vi "Run.vi"(8 "error in (no error)":errorcluster, 10 "OTP Cluster Out":T1, 11 "Harmonics in":refnum<class "Harmonics.lvclass">) -> (0 "error out":errorcluster, 1 "Parameters":cluster{"Name":string, "Value":string}[](array[cluster]), 2 "Canceled":bool, 3 "Harmonics out":refnum<class "Harmonics.lvclass">)   [LabVIEW 2020, in "Harmonics.lvclass"]
doc: "This is the main test vi. It is here that the test is implemented."
uses:
  Harmonics.lvclass
  Controls/Run states.ctl
  Instruments/Spectrum Analyzer/Spectrum Analyzer.lvclass
  Measurement.lvclass
  Devices/Controls/Change setting mode enum.ctl
  Devices/PIC-device/PIC-Device.lvclass
  Controls/Loop order.ctl
  XML Handler/XML Handler.lvclass
  Support VI/Update parameters (single).vi
  Instruments/Power Supply/Power Supply.lvclass
  Support VI/Update parameters (array).vi
  Instruments/Digital Multimeter/Digital Multimeter.lvclass
  Devices/Device.lvclass
  Path Control/PathControl.lvclass
  Path Control/Paths.ctl
  Instruments/Power Meter/Power Meter.lvclass
  Instruments/Signal Generator/Signal Generator.lvclass
  C:/Sandbox/Git_Sandbox/WiSpry Test Framework source code (LV20)/WiSpry Test Framework/Measurements/Measurement.lvclass
  Controls/OTP_Cluster.ctl
panel:
  out "Power Meter reading (dBm)":dbl[](array[numeric])
  out "Parameters":string
  out "Current Power [dBm]":dbl
  out "Current Frequency [Hz]":dbl format="%#_6p"
  out "Progress":u8(slide) scale=0.0..100.0
  in  "Cancel Button":bool
  out "XY Graph":cluster{dbl[], dbl[]}[](graph)
  out "Estimated finish time":timestamp format="%<%X>T"
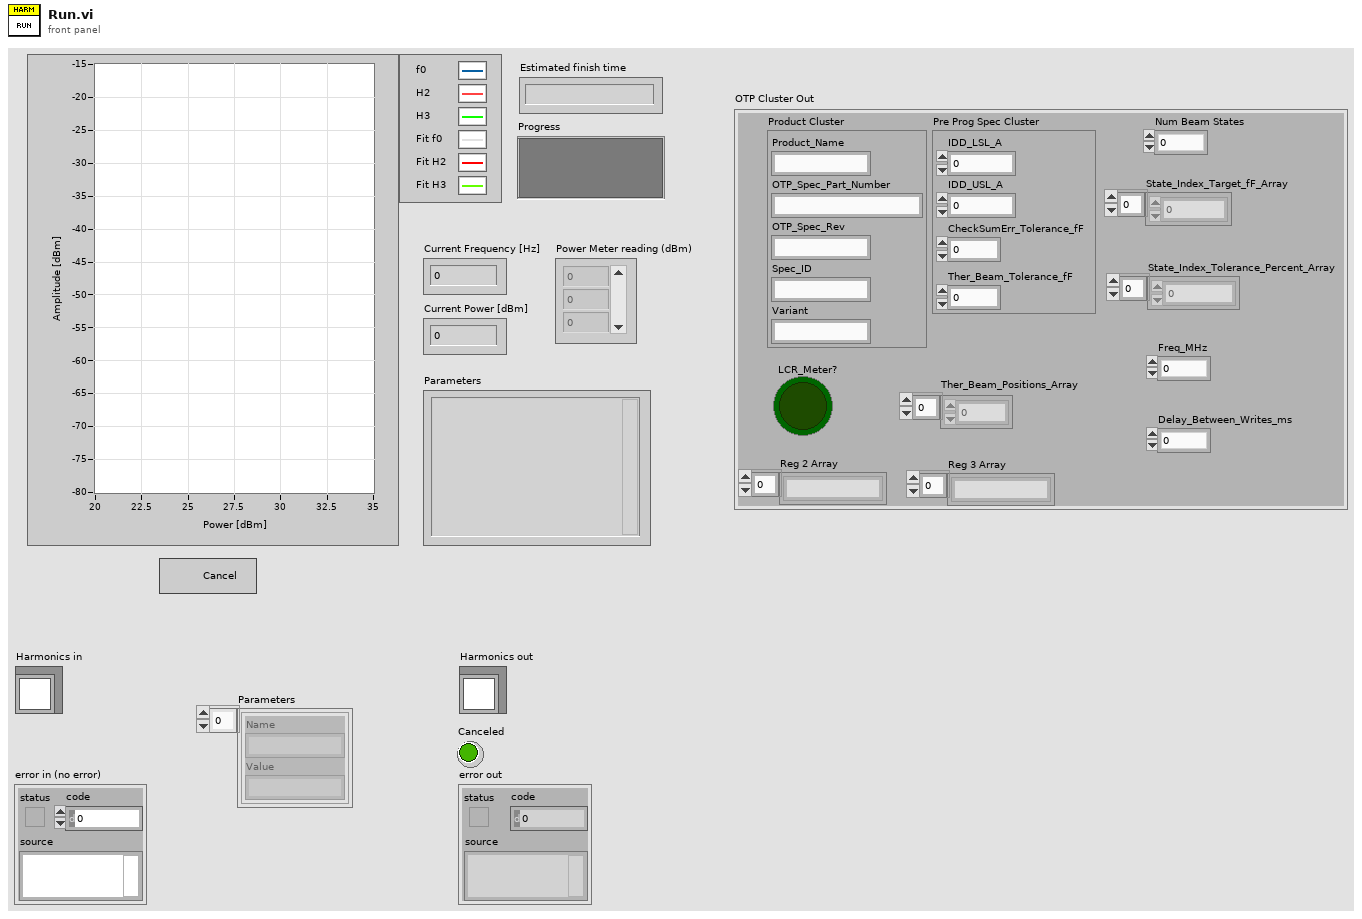
[diagram p1: front panel]
types:
  T1 = typedef "OTP_Cluster.ctl" = cluster{"Product Cluster":cluster{"Product_Name":string, "OTP_Spec_Part_Number":string, "OTP_Spec_Rev":string, "Spec_ID":string, "Variant":string}, "Pre Prog Spec Cluster":cluster{"IDD_LSL_A":dbl, "IDD_USL_A":dbl, "CheckSumErr_Tolerance_fF":dbl, "Ther_Beam_Tolerance_fF":dbl}, "LCR_Meter?":bool, "Reg 2 Array":string[], "Reg 3 Array":string[], "Num Beam States":i32, "State_Index_Target_fF_Array":dbl[], "State_Index_Tolerance_Percent_Array":dbl[], "Freq_MHz":dbl, "Delay_Between_Writes_ms":i32, "Ther_Beam_Positions_Array":i8[]}
  T2 = typedef "Harmonics.lvclass/Loop order.ctl" = enum16{"Device -> Power -> Frequency", "Device -> Frequency -> Power"}
  T3 = typedef "Harmonics.lvclass/Run states.ctl" = enum16{"Init", "Set Device", "Set Power", "Set Frequency", "Read Environment", "Measure", "Done"}
  T4 = typedef "PIC-Device.lvclass/Change setting mode enum.ctl" = enum16{"Init", "Next", "Reset"}
  T5 = typedef "PathControl.lvclass/Paths.ctl" = enum16{"SigGen 1 -> DUT", "SigGen 2 -> DUT", "SigGen 1 -> PM 1", "SigGen 1 -> PM 2", "DUT -> SA", "DUT -> PM 2", "VSG -> DUT", "SigGen 2 -> PM 1", "SigGen 2 -> PM 2"}
  T6 = typedef "Harmonics.lvclass/Config info.ctl" = cluster{"RBW":dbl, "VBW ":dbl, "Number of Averages":i32, "Average On":bool, "Symbols":i32[], "All Harm":bool, "Loop order":T2, "Power Window":dbl, "Frequency (MHz)":string, "Power (dBm)":string, "PM for power leveling":u8, "Zero span":bool, "Stop level":dbl}
  T7 = typedef "XML Handler.lvclass/Result Cluster.ctl" = cluster{"Name":string, "Value":string}
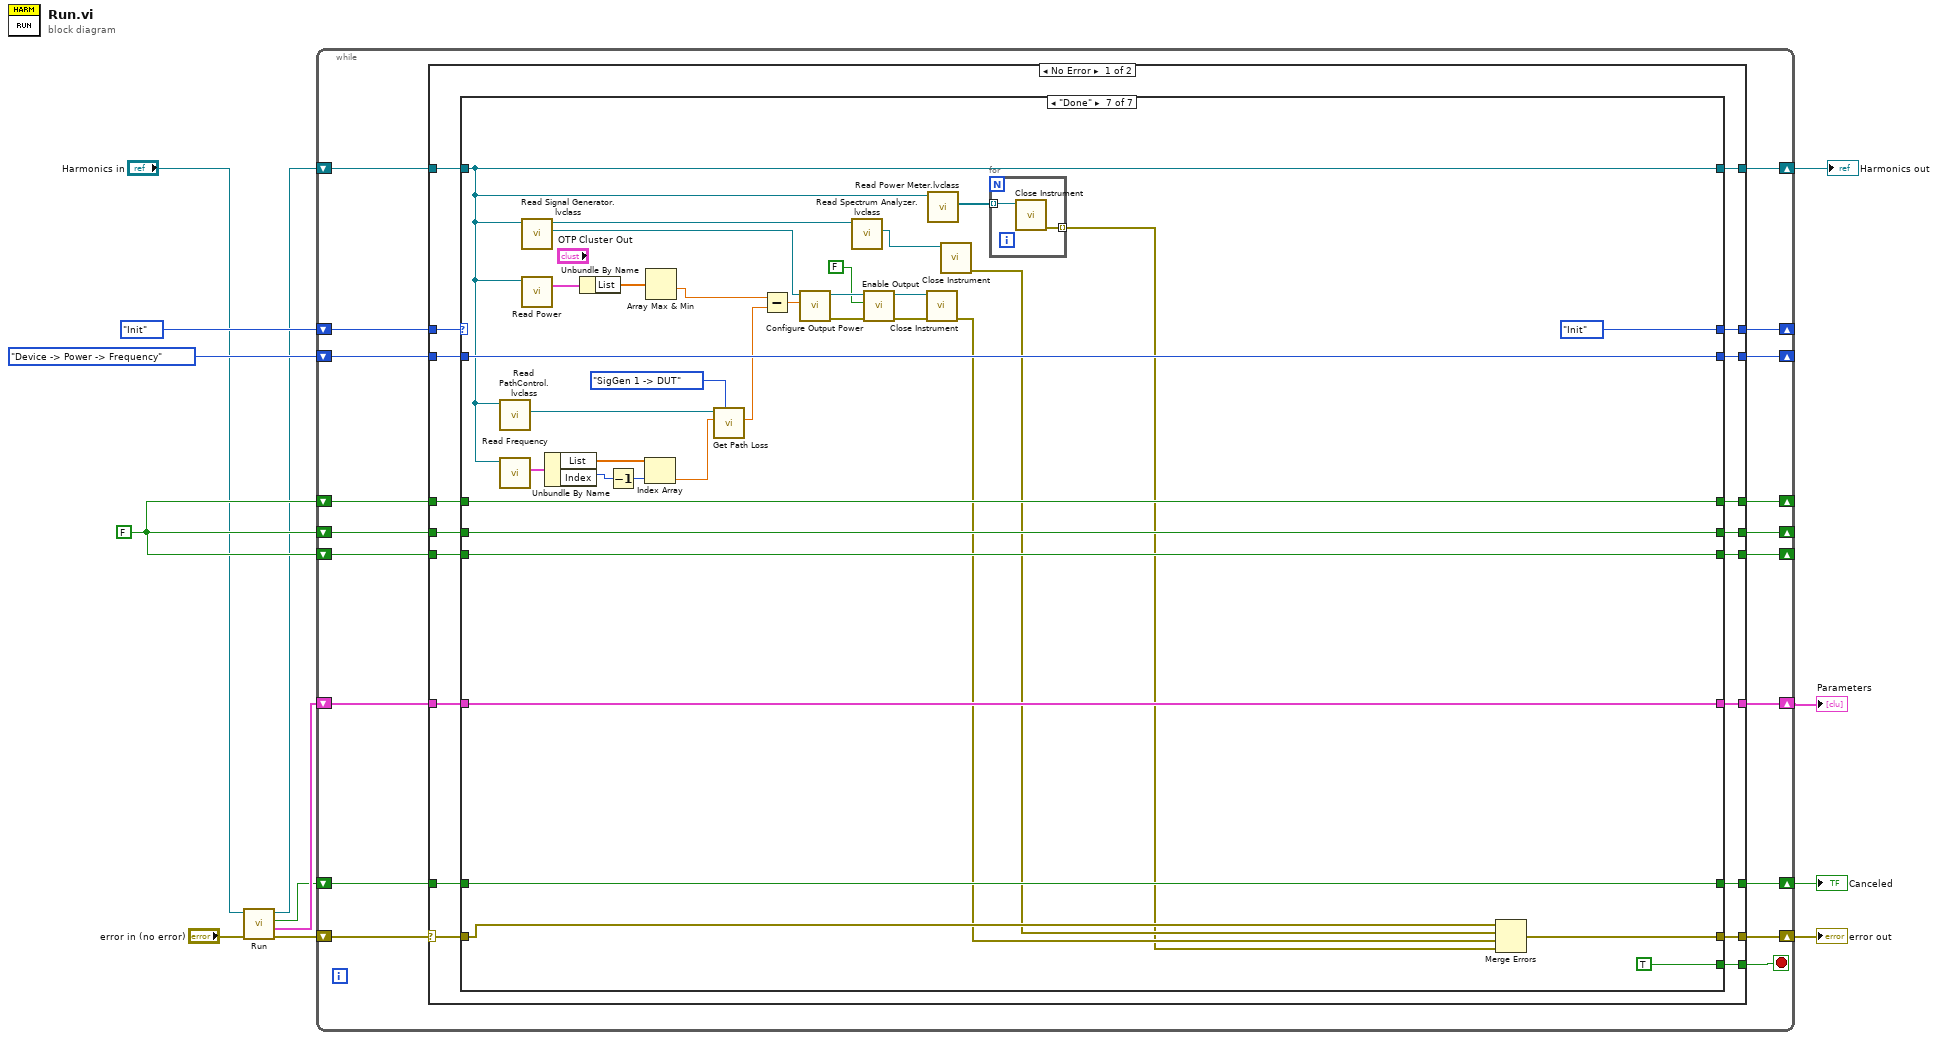
[diagram p0: block diagram]
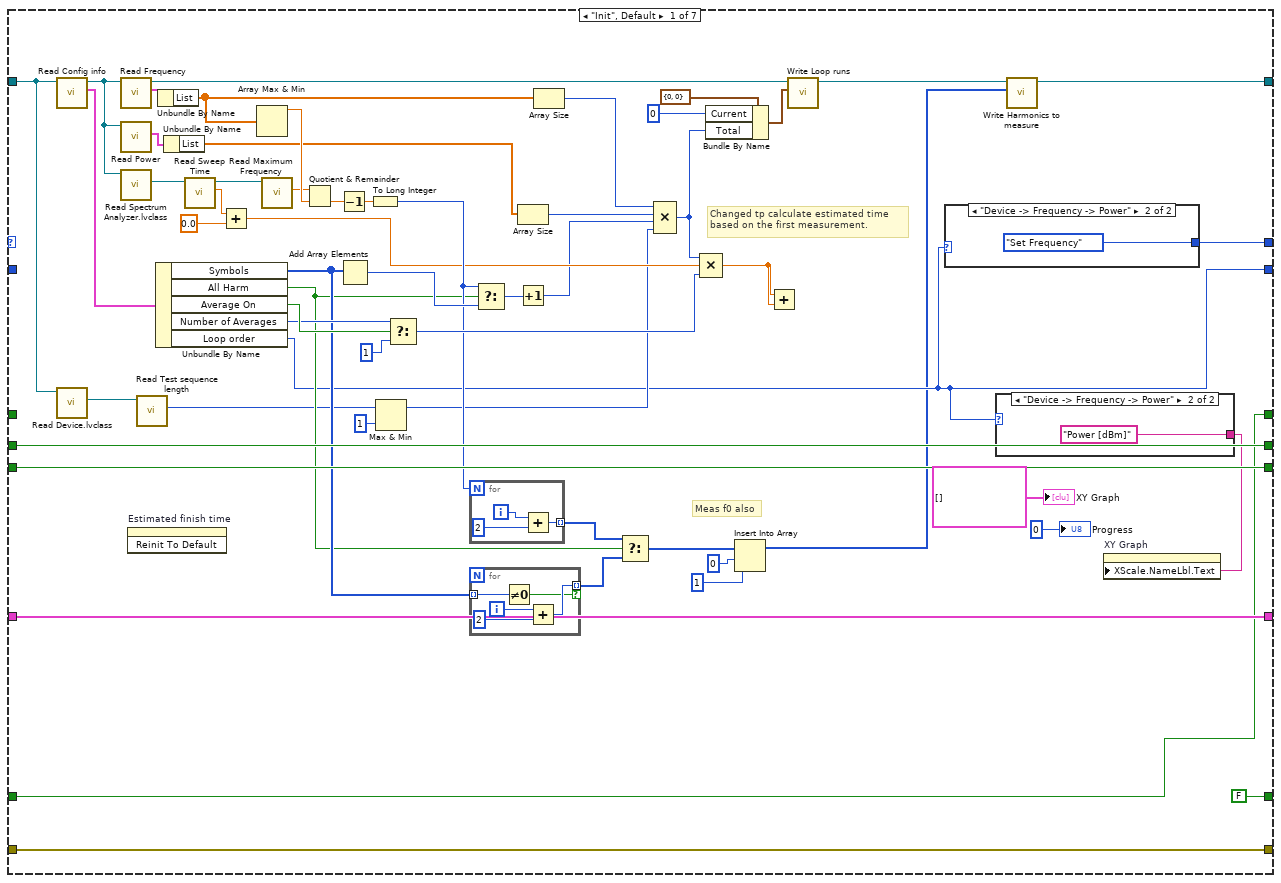
[diagram p2: hidden frame]
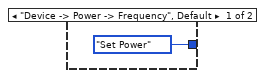
[diagram p3: hidden frame]
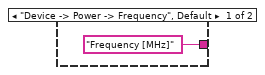
[diagram p4: hidden frame]
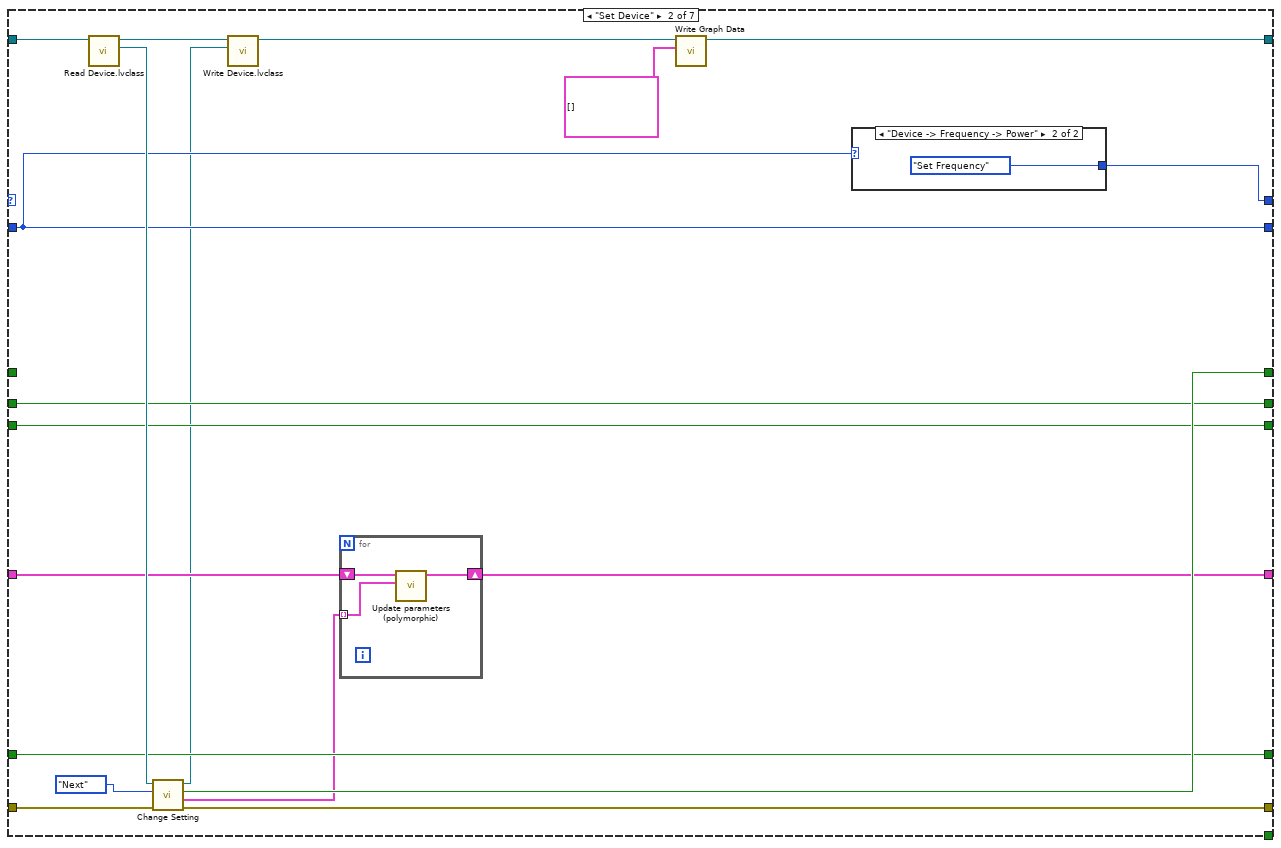
[diagram p5: hidden frame]
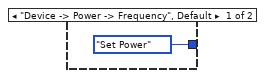
[diagram p6: hidden frame]
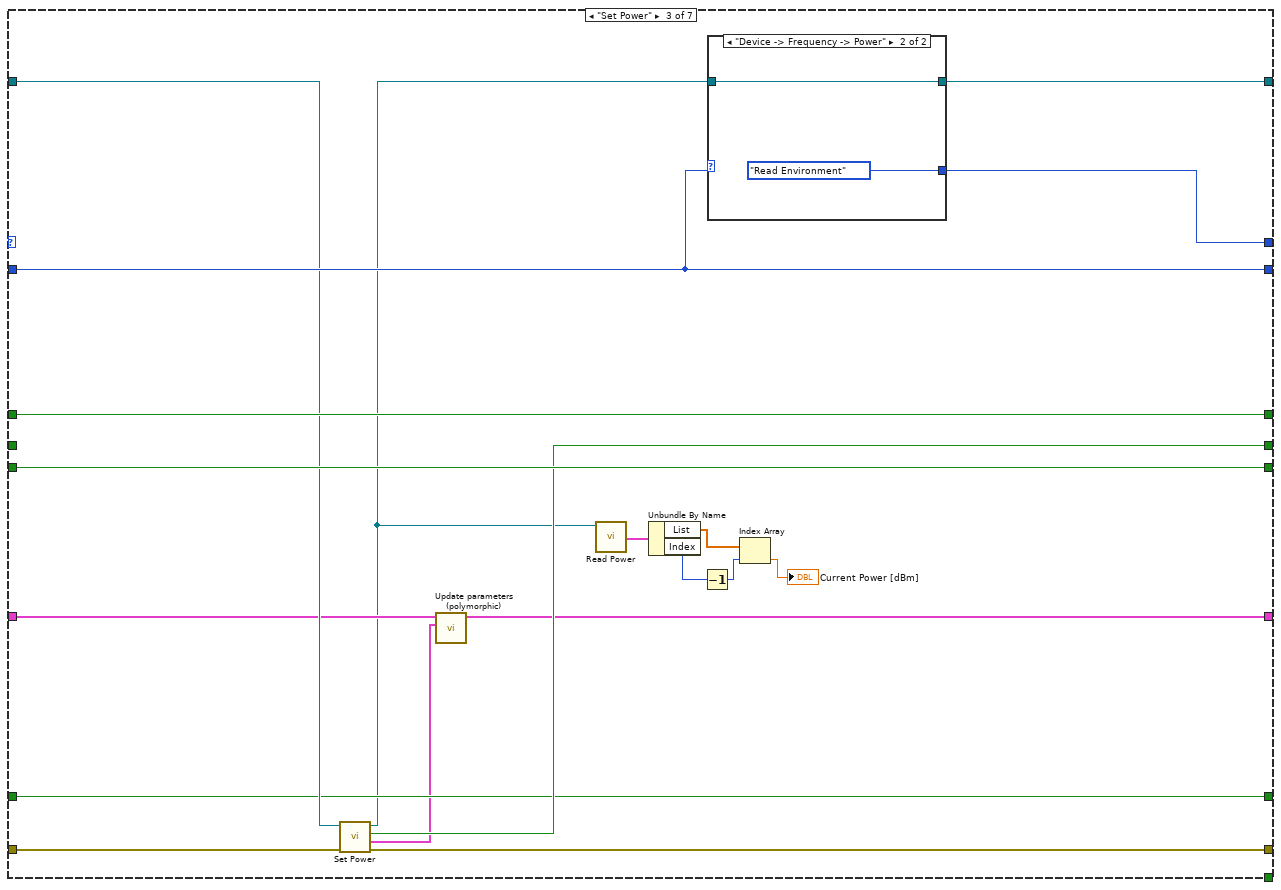
[diagram p7: hidden frame]
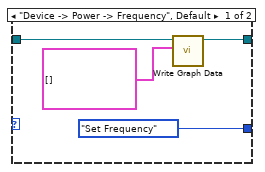
[diagram p8: hidden frame]
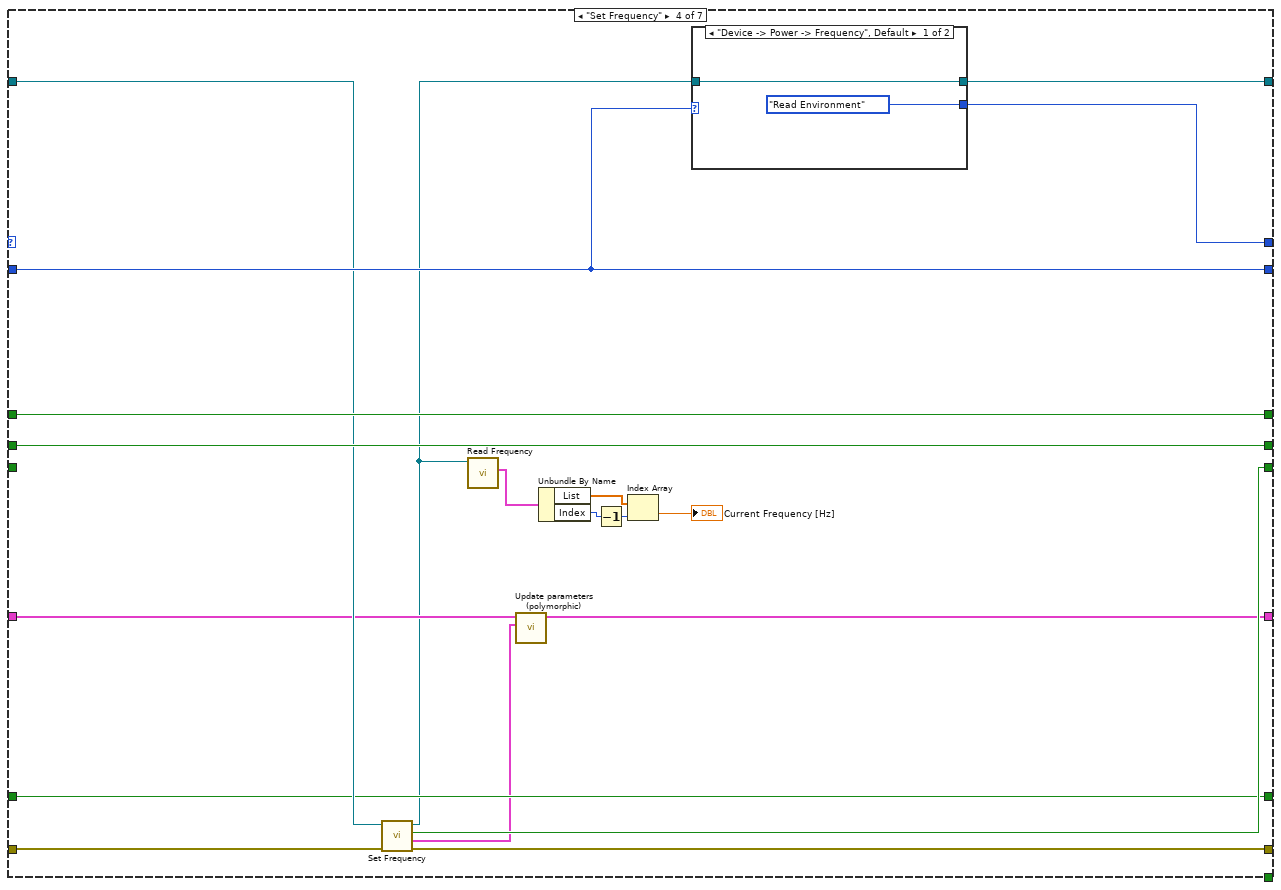
[diagram p9: hidden frame]
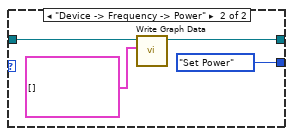
[diagram p10: hidden frame]
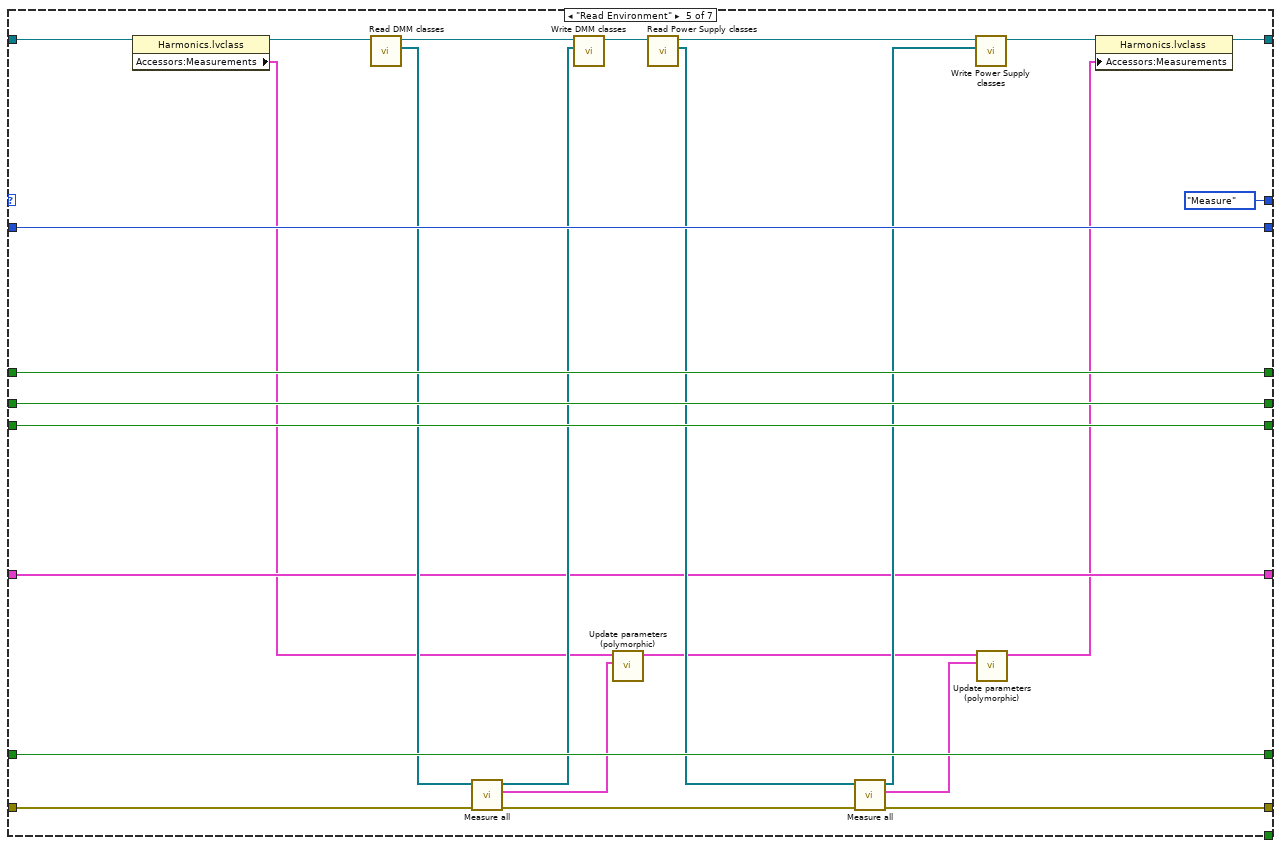
[diagram p11: hidden frame]
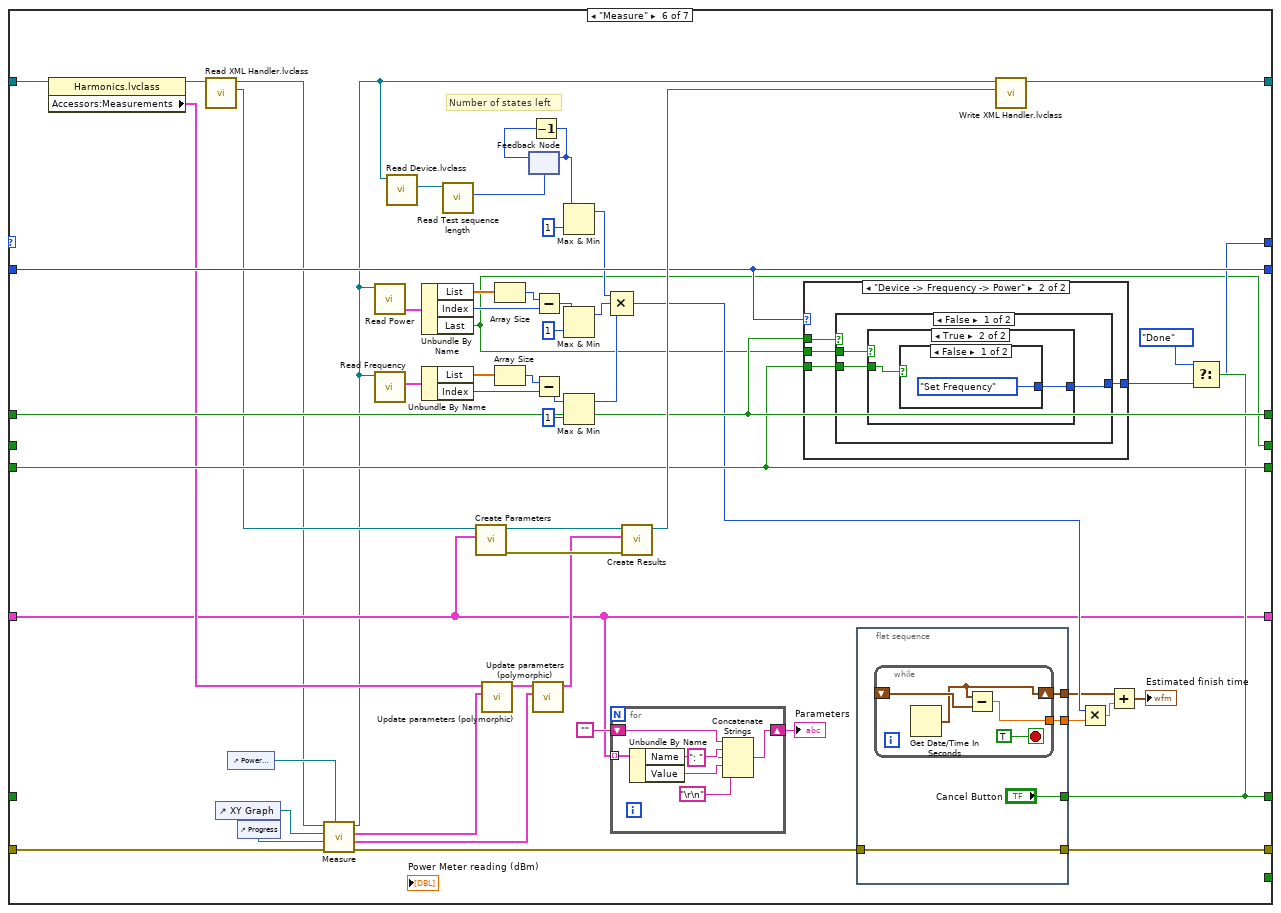
[diagram p12: hidden frame]
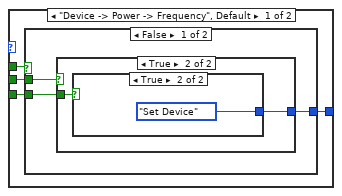
[diagram p13: hidden frame]
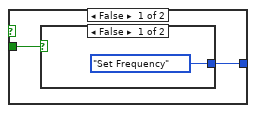
[diagram p14: hidden frame]
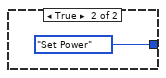
[diagram p15: hidden frame]
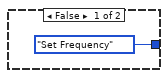
[diagram p16: hidden frame]
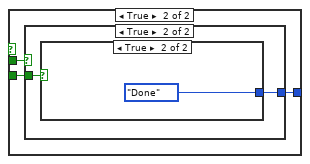
[diagram p17: hidden frame]
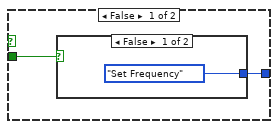
[diagram p18: hidden frame]
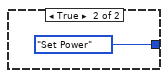
[diagram p19: hidden frame]
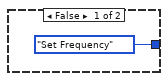
[diagram p20: hidden frame]
diagram:
  w10 = FALSE
  n1 = call-parent "Run.vi"("error in (no error)"="error in (no error)", "Measurements in"="Harmonics in") -> ("error out"=w5:errorcluster, "Parameters"=w3:cluster{"Name":string, "Value":string}[], "Canceled"=w2:bool, "Measurements out"=w1:refnum<class "Harmonics.lvclass">)  [unwired: 5 in, 1 out]
  n2 = while {
    shift-right: [w29] -> w12
    shift-left: w5 -> [w15]
    shift-right: [w31] -> w13
    shift-left: w1 -> [w14]
    shift-right: [w26] -> _
    shift-left: Run_states."Init" ("Run states") -> [w32]
    shift-right: [w28] -> _
    shift-left: w10 -> [w27]
    shift-right: [w25] -> _
    shift-left: Loop_order."Device -> Power -> Frequency" ("Loop order") -> [w24]
    shift-right: [w21] -> _
    shift-left: w10 -> [w23]
    shift-right: [w20] -> _
    shift-left: w10 -> [w22]
    shift-right: [w19] -> w8
    shift-left: w2 -> [w18]
    shift-right: [w16] -> w7
    shift-left: w3 -> [w17]
    stop <- w30 stop-if-true
    n3 = case shown="No Error" w15 {
      selector: w15 -> [w48 w376]
      tunnel: w14 -> [w51 w377]
      tunnel: w32 -> [w50 _]
      tunnel: [w49 w377] -> w31
      tunnel: [w47 TRUE] -> w30
      tunnel: [w46 w376] -> w29
      tunnel: [w45 _] -> w28
      tunnel: w27 -> [w44 _]
      tunnel: [w43 _] -> w26
      tunnel: [w42 _] -> w25
      tunnel: w24 -> [w41 _]
      tunnel: w23 -> [w40 _]
      tunnel: w22 -> [w39 _]
      tunnel: [w38 _] -> w21
      tunnel: [w37 _] -> w20
      tunnel: [w36 _] -> w19
      tunnel: w18 -> [w35 _]
      tunnel: w17 -> [w34 w375]
      tunnel: [w33 w375] -> w16
      frame No Error {
        n4 = case shown="\"Done\"" w50 {
          tunnel: w51 -> [w94 w139 w158 w183 w199 w223 w342]
          tunnel: [w83 w128 w155 w180 w200 w274 w342] -> w49
          tunnel: w48 -> [w69 w136 w159 w184 w205 w238 w360]
          tunnel: [_ _ _ _ _ _ TRUE] -> w47
          tunnel: [w69 w125 w154 w179 w204 w272 w357] -> w46
          tunnel: [w60 w135 w163 w188 w220 w270 w371] -> w45
          tunnel: w44 -> [_ _ w163 w188 w220 w270 w371]
          tunnel: [w62 w131 w161 w186 Run_states."Measure" ("Run states") w265 Run_states."Init" ("Run states")] -> w43
          tunnel: [w61 w132 w162 w187 w219 w271 w372] -> w42
          tunnel: w41 -> [_ w132 w162 w187 w219 w271 w372]
          tunnel: w40 -> [w90 w134 _ w185 w218 _ w370]
          tunnel: w39 -> [w89 w133 w160 _ w217 w269 w369]
          tunnel: [w90 w134 w157 w185 w218 w221 w370] -> w38
          tunnel: [w89 w133 w160 w182 w217 w269 w369] -> w37
          tunnel: [FALSE ("Last setting") w130 w156 w181 w216 w268 w366] -> w36
          tunnel: w35 -> [w60 w130 w156 w181 w216 _ w366]
          tunnel: w34 -> [w73 w124 w153 w178 w197 w225 w365]
          tunnel: [w73 w122 w152 w177 w197 w225 w365] -> w33
          frame "Init", Default {
            # "Changed tp calculate estimated time \nbased on the first measurement."
            # "Meas f0 also"
            n5 = call "Read Config info.vi"("Harmonics in"=w94) -> ("Config info"=w107:T6, "Harmonics out"=w108:refnum<class "Harmonics.lvclass">)  [unwired: 9 in]
            n6 = call "Read Device.lvclass.vi"("Measurements in"=w94) -> ("Device.lvclass"=w91:refnum<class "Device.lvclass">)  [unwired: 9 in, 1 out]
            n7 = call "Read Frequency.vi"("Harmonics in"=w108) -> ("Frequency"=w82:cluster{"List":dbl[], "Index":i32, "Last":bool}, "Harmonics out"=w78:refnum<class "Harmonics.lvclass">)  [unwired: 9 in]
            n8 = call "Read Power.vi"("Harmonics in"=w108) -> ("Power"=w80:cluster{"List":dbl[], "Index":i32, "Last":bool})  [unwired: 9 in, 1 out]
            n9 = call "Read Spectrum Analyzer.lvclass.vi"("Harmonics in"=w108) -> ("Spectrum Analyzer.lvclass"=w105:refnum<class "Spectrum Analyzer.lvclass">)  [unwired: 9 in, 1 out]
            n10 = invoke on="Estimated finish time" class="AbsTime (strict)" method="Reinit To Default"() -> ()  [unwired: 3 in, 3 out]
            n11 = call-dynamic "Read Test sequence length.vi"("Device in"=w91) -> ("Test sequence length"=w65:i32)  [unwired: 8 in, 2 out]
            n12 = Unbundle By Name(w107) -> ("Symbols"=w87:i32[], "All Harm"=w84:bool, "Average On"=w99:bool, "Number of Averages"=w98:i32, "Loop order"=w61:T2)
            n13 = Unbundle By Name(w82) -> ("List"=w81:dbl[])
            n14 = Unbundle By Name(w80) -> ("List"=w79:dbl[])
            n15 = call "Read Sweep Time.vi"("Spectrum Analyzer in"=w105) -> ("Sweep Time"=w100:dbl, "Spectrum Analyzer out"=w104:refnum<class "Spectrum Analyzer.lvclass">)  [unwired: 9 in]
            n16 = Add(x=w100, y=0.0) -> (x+y=w67:dbl)
            n17 = Array Max & Min(array=w81) -> (max value=w103:dbl)  [unwired: 3 out]
            n18 = call "Read Maximum Frequency.vi"("Spectrum Analyzer in"=w104) -> ("Maximum Frequency"=w102:dbl)  [unwired: 9 in, 1 out]
            n19 = Quotient & Remainder(x=w102, y=w103) -> (floor(x/y)=w101:dbl)  [unwired: 1 out]
            n20 = Decrement(x=w101) -> (x-1=w95:dbl)
            n21 = Add Array Elements(numeric array=w87) -> (sum=w106:i32)
            n22 = To Long Integer(number=w95) -> (32bit integer=w88:i32)
            n23 = Max & Min(x=w65, y=1) -> (max(x,y)=w64:i32)  [unwired: 1 out]
            n24 = Select(t=w98, s=w99, f=1) -> (s? t:f=w96:i32)
            n25 = for {
              N: w88 -> [_]
              tunnel: [w118] -> w86 mode=indexing
              i -> [w120]
              n26 = Add(x=w120, y=2) -> (x+y=w118:i32)
            }
            n27 = for {
              tunnel: w87 -> [w114] mode=indexing
              tunnel: [w115] -> w85 mode=indexing if=w113
              i -> [w117]
              n28 = Not Equal To 0?(x=w114) -> (x != 0?=w113:bool)
              n29 = Add(x=w117, y=2) -> (x+y=w115:i32)
            }
            n30 = Select(t=w88, s=w84, f=w106) -> (s? t:f=w54:i32)
            n31 = Array Size(array=w79) -> (size(s)=w92:i32)
            n32 = Increment(x=w54) -> (x+1=w53:i32)
            n33 = Array Size(array=w81) -> (size(s)=w93:i32)
            n34 = Select(t=w86, s=w84, f=w85) -> (s? t:f=w58:i32[])
            n35 = Compound Arithmetic op=MULTIPLY(w93, w92, w53, w64) -> (w74:i32)
            n36 = Compound Arithmetic op=MULTIPLY(w74, w67, w96) -> (w52:dbl)
            n37 = Bundle By Name(cluster=cluster{"Current":u32, "Total":u32} {"Current"=0, "Total"=0} ("Loop runs"), "Current"=u32 0, "Total"=w74) -> (w75:cluster{"Current":u32, "Total":u32})
            n38 = Insert Into Array(array=w58, index=0, new element=1 ("new element/subarray")) -> (w57:i32[])
            n39 = Add(x=w52, y=w52) -> ()  [unwired: 1 out]
            n40 = call "Write Loop runs.vi"("Loop runs"=w75, "Measurements in"=w78) -> ("Measurements out"=w68:refnum<class "Harmonics.lvclass">)  [unwired: 9 in]
            n41 = case shown="\"Device -> Frequency -> Power\"" w61 {
              tunnel: [Run_states."Set Power" ("Run states") Run_states."Set Frequency" ("Run states")] -> w62
              frame "Device -> Power -> Frequency", Default {
              }
              frame "Device -> Frequency -> Power" {
              }
            }
            n42 = case shown="\"Device -> Frequency -> Power\"" w61 {
              tunnel: ["Frequency [MHz]" "Power [dBm]"] -> w70
              frame "Device -> Power -> Frequency", Default {
              }
              frame "Device -> Frequency -> Power" {
              }
            }
            n43 = call "Write Harmonics to measure.vi"("Harmonics to measure"=w57, "Harmonics in"=w68) -> ("Harmonics out"=w83:refnum<class "Harmonics.lvclass">)  [unwired: 9 in]
            n44 = property on="XY Graph" class="XYGraph (strict)"("XScale.NameLbl.Text"=w70) -> ()  [unwired: 2 in, 2 out]
            "XY Graph" <- cluster{dbl[], dbl[]}[] [] ("XY Graph")
            "Progress" <- u8 0 ("Progress")
          }
          frame "Set Device" {
            n45 = call "Read Device.lvclass.vi"("Measurements in"=w139) -> ("Device.lvclass"=w138:refnum<class "Device.lvclass">, "Measurements out"=w129:refnum<class "Harmonics.lvclass">)  [unwired: 9 in]
            n46 = call-dynamic "Change Setting.vi"("error in (no error)"=w136, "Change setting mode"=Change_setting_mode_enum."Next", "Device in"=w138) -> ("error out"=w125:errorcluster, "Changes"=w123:cluster{"Name":string, "Value":string}[], "Last setting"=w135:bool, "Device out"=w121:refnum<class "Device.lvclass">)  [unwired: 5 in]
            n47 = call "Write Device.lvclass.vi"("Device.lvclass"=w121, "Measurements in"=w129) -> ("Measurements out"=w126:refnum<class "Harmonics.lvclass">)  [unwired: 9 in]
            n48 = for {
              shift-right: [w141] -> w122
              shift-left: w124 -> [w142]
              tunnel: w123 -> [w140] mode=indexing
              n49 = call-poly "Update parameters (polymorphic).vi"("New Parameter"=w140, "Parameters"=w142) -> ("Parameters Out"=w141:cluster{"Name":string, "Value":string}[])  [unwired: 9 in]
            }
            n50 = call "Write Graph Data.vi"("Graph Data"=cluster{"Array":dbl[], "Array":dbl[]}[] [], "Harmonics in"=w126) -> ("Harmonics out"=w128:refnum<class "Harmonics.lvclass">)  [unwired: 9 in]
            n51 = case shown="\"Device -> Frequency -> Power\"" w132 {
              tunnel: [Run_states."Set Power" ("Run states") Run_states."Set Frequency" ("Run states")] -> w131
              frame "Device -> Power -> Frequency", Default {
              }
              frame "Device -> Frequency -> Power" {
              }
            }
          }
          frame "Set Power" {
            n52 = call "Set Power.vi"("error in (no error)"=w159, "Harmonics in"=w158) -> ("error out"=w154:errorcluster, "Parameter"=w151:cluster{"Name":string, "Value":string}, "Last Power?"=w157:bool, "Harmonics out"=w150:refnum<class "Harmonics.lvclass">)  [unwired: 6 in]
            n53 = call-poly "Update parameters (polymorphic).vi"("New Parameter"=w151, "Parameters"=w153) -> ("Parameters Out"=w152:cluster{"Name":string, "Value":string}[])  [unwired: 9 in]
            n54 = call "Read Power.vi"("Harmonics in"=w150) -> ("Power"=w149:cluster{"List":dbl[], "Index":i32, "Last":bool})  [unwired: 9 in, 1 out]
            n55 = Unbundle By Name(w149) -> ("List"=w147:dbl[], "Index"=w145:i32)
            n56 = Decrement(x=w145) -> (x-1=w146:i32)
            n57 = case shown="\"Device -> Frequency -> Power\"" w162 {
              tunnel: [Run_states."Set Frequency" ("Run states") Run_states."Read Environment" ("Run states")] -> w161
              tunnel: w150 -> [w166 w168]
              tunnel: [w165 w168] -> w155
              frame "Device -> Power -> Frequency", Default {
                n58 = call "Write Graph Data.vi"("Graph Data"=cluster{"Array":dbl[], "Array":dbl[]}[] [], "Harmonics in"=w166) -> ("Harmonics out"=w165:refnum<class "Harmonics.lvclass">)  [unwired: 9 in]
              }
              frame "Device -> Frequency -> Power" {
              }
            }
            n59 = Index Array(array=w147, index=w146) -> (element=→"Current Power [dBm]":dbl)
          }
          frame "Set Frequency" {
            n60 = call "Set Frequency.vi"("error in (no error)"=w184, "Harmonics in"=w183) -> ("error out"=w179:errorcluster, "Parameter"=w176:cluster{"Name":string, "Value":string}, "Last Frequency?"=w182:bool, "Harmonics out"=w175:refnum<class "Harmonics.lvclass">)  [unwired: 6 in]
            n61 = call "Read Frequency.vi"("Harmonics in"=w175) -> ("Frequency"=w174:cluster{"List":dbl[], "Index":i32, "Last":bool})  [unwired: 9 in, 1 out]
            n62 = call-poly "Update parameters (polymorphic).vi"("New Parameter"=w176, "Parameters"=w178) -> ("Parameters Out"=w177:cluster{"Name":string, "Value":string}[])  [unwired: 9 in]
            n63 = Unbundle By Name(w174) -> ("List"=w173:dbl[], "Index"=w172:i32)
            n64 = Decrement(x=w172) -> (x-1=w171:i32)
            n65 = Index Array(array=w173, index=w171) -> (element=→"Current Frequency [Hz]":dbl)
            n66 = case shown="\"Device -> Power -> Frequency\", Default" w187 {
              tunnel: [Run_states."Read Environment" ("Run states") Run_states."Set Power" ("Run states")] -> w186
              tunnel: [w189 w192] -> w180
              tunnel: w175 -> [w189 w193]
              frame "Device -> Power -> Frequency", Default {
              }
              frame "Device -> Frequency -> Power" {
                n67 = call "Write Graph Data.vi"("Graph Data"=cluster{"Array":dbl[], "Array":dbl[]}[] [], "Harmonics in"=w193) -> ("Harmonics out"=w192:refnum<class "Harmonics.lvclass">)  [unwired: 9 in]
              }
            }
          }
          frame "Read Environment" {
            n68 = property class="Harmonics.lvclass"(reference=w199) -> (reference out=w198:refnum<class "Harmonics.lvclass">, "Accessors:Measurements"=w196:cluster{"Name":string, "Value":string}[])  [unwired: 1 in, 1 out]
            n69 = call-dynamic "Read DMM classes.vi"("Measurements in"=w198) -> ("DMM classes"=w210:refnum<class "Digital Multimeter.lvclass">[], "Measurements out"=w215:refnum<class "Harmonics.lvclass">)  [unwired: 9 in]
            n70 = call "Measure all.vi"("error in (no error)"=w205, "Digital Multimeters in"=w210) -> ("error out"=w208:errorcluster, "Measurements"=w207:T7[], "Digital Multimeters out"=w209:refnum<class "Digital Multimeter.lvclass">[])  [unwired: 5 in, 2 out]
            n71 = call-dynamic "Write DMM classes.vi"("DMM classes"=w209, "Measurements in"=w215) -> ("Measurements out"=w212:refnum<class "Harmonics.lvclass">)  [unwired: 9 in]
            n72 = call-poly "Update parameters (polymorphic).vi"("New Parameters"=w207, "Parameters"=w196) -> ("Parameters Out"=w206:cluster{"Name":string, "Value":string}[])  [unwired: 9 in]
            n73 = call-dynamic "Read Power Supply classes.vi"("Measurements in"=w212) -> ("Power Supply classes"=w214:refnum<class "Power Supply.lvclass">[], "Measurements out"=w202:refnum<class "Harmonics.lvclass">)  [unwired: 9 in]
            n74 = call "Measure all.vi"("error in (no error)"=w208, "Power Supplies in"=w214) -> ("error out"=w204:errorcluster, "Measurements"=w211:T7[], "Power Supplies out"=w213:refnum<class "Power Supply.lvclass">[])  [unwired: 5 in, 2 out]
            n75 = call-dynamic "Write Power Supply classes.vi"("Power Supply classes"=w213, "Measurements in"=w202) -> ("Measurements out"=w201:refnum<class "Harmonics.lvclass">)  [unwired: 9 in]
            n76 = call-poly "Update parameters (polymorphic).vi"("New Parameters"=w211, "Parameters"=w206) -> ("Parameters Out"=w195:cluster{"Name":string, "Value":string}[])  [unwired: 9 in]
            n77 = property class="Harmonics.lvclass"(reference=w201, "Accessors:Measurements"=w195) -> (reference out=w200:refnum<class "Harmonics.lvclass">)  [unwired: 1 in, 1 out]
          }
          frame "Measure" {
            # "Number of states left"
            n78 = property class="Harmonics.lvclass"(reference=w223) -> (reference out=w260:refnum<class "Harmonics.lvclass">, "Accessors:Measurements"=w259:cluster{"Name":string, "Value":string}[])  [unwired: 1 in, 1 out]
            n79 = call "Read XML Handler.lvclass.vi"("Measurements in"=w260) -> ("XML Handler.lvclass"=w263:refnum<class "XML Handler.lvclass">, "Measurements out"=w224:refnum<class "Harmonics.lvclass">)  [unwired: 9 in]
            n80 = control-ref of="XY Graph"() -> (w275:refnum<vi>)
            n81 = control-ref of="Power Meter reading (dBm)"() -> (w254:refnum<vi>)
            n82 = control-ref of="Progress"() -> (w264:refnum<vi>)
            n83 = call "Measure.vi"("Power Meter reading reference"=w254, "error in (no error)"=w238, "Progress Ref"=w264, "XY Graph Reference"=w275, "Harmonics in"=w224) -> ("error out"=w273:errorcluster, "Cal values"=w257:cluster{"Name":string, "Value":string}[], "Results"=w258:T7[], "Harmonics out"=w222:refnum<class "Harmonics.lvclass">)  [unwired: 3 in]
            n84 = call "Read Power.vi"("Harmonics in"=w222) -> ("Power"=w250:cluster{"List":dbl[], "Index":i32, "Last":bool})  [unwired: 9 in, 1 out]
            n85 = call "Read Frequency.vi"("Harmonics in"=w222) -> ("Frequency"=w249:cluster{"List":dbl[], "Index":i32, "Last":bool})  [unwired: 9 in, 1 out]
            n86 = call "Read Device.lvclass.vi"("Measurements in"=w222) -> ("Device.lvclass"=w253:refnum<class "Device.lvclass">)  [unwired: 9 in, 1 out]
            n87 = Unbundle By Name(w250) -> ("List"=w248:dbl[], "Index"=w246:i32, "Last"=w221:bool)
            n88 = Unbundle By Name(w249) -> ("List"=w245:dbl[], "Index"=w244:i32)
            n89 = call-dynamic "Read Test sequence length.vi"("Device in"=w253) -> ("Test sequence length"=w251:i32)  [unwired: 8 in, 2 out]
            n90 = call "Create Parameters.vi"("Parameters"=w225, "XML Handler in"=w263) -> ("error out"=w261:errorcluster, "XML Handler out"=w262:refnum<class "XML Handler.lvclass">)  [unwired: 8 in]
            n91 = call-poly "Update parameters (polymorphic).vi"("New Parameters"=w258, "Parameters"=w259) -> ("Parameters Out"=w256:cluster{"Name":string, "Value":string}[])  [unwired: 9 in]
            n92 = Array Size(array=w248) -> (size(s)=w247:i32)
            n93 = Array Size(array=w245) -> (size(s)=w235:i32)
            n94 = feedback #1(w251) -> (w252:i32)
            n95 = Decrement(x=w252) -> (x-1=w233:i32)
            n96 = feedback-in #1(w233) -> ()
            n97 = call-poly "Update parameters (polymorphic).vi"("New Parameters"=w257, "Parameters"=w256) -> ("Parameters Out"=w255:cluster{"Name":string, "Value":string}[])  [unwired: 9 in]
            n98 = Subtract(x=w247, y=w246) -> (x-y=w230:i32)
            n99 = Subtract(x=w235, y=w244) -> (x-y=w234:i32)
            n100 = Max & Min(x=w233, y=1) -> (max(x,y)=w231:i32)  [unwired: 1 out]
            n101 = Max & Min(x=w230, y=1) -> (max(x,y)=w229:i32)  [unwired: 1 out]
            n102 = Max & Min(x=w234, y=1) -> (max(x,y)=w228:i32)  [unwired: 1 out]
            n103 = Compound Arithmetic op=MULTIPLY(w231, w229, w228) -> (w243:i32)
            n104 = for {
              tunnel: w225 -> [w283] mode=indexing
              shift-right: [w277] -> w227
              shift-left: "" -> [w282]
              n105 = Unbundle By Name(w283) -> ("Name"=w281:string, "Value"=w279:string)
              n106 = Concatenate Strings(w282, w281, ": " ("string"), w279, "\r\n") -> (w277:string)
            }
            "Parameters" <- w227
            n107 = call "Create Results.vi"("error in (no error)"=w261, "Results"=w255, "XML Handler in"=w262) -> ("XML Handler out"=w276:refnum<class "XML Handler.lvclass">)  [unwired: 7 in, 1 out]
            n108 = case shown="\"Device -> Frequency -> Power\"" w271 {
              tunnel: w270 -> [w287 w313]
              tunnel: w221 -> [w286 w312]
              tunnel: w269 -> [w285 w311]
              tunnel: [w284 w310] -> w267
              frame "Device -> Power -> Frequency", Default {
                n109 = case shown="False" w287 {
                  tunnel: w286 -> [w290 w301]
                  tunnel: w285 -> [w289 w300]
                  tunnel: [w288 w299] -> w284
                  frame False {
                    n110 = case shown="True" w290 {
                      tunnel: w289 -> [w292 w296]
                      tunnel: [w291 w295] -> w288
                      frame False {
                        n111 = case shown="False" w292 {
                          tunnel: [Run_states."Set Frequency" ("Run states") Run_states."Set Power" ("Run states")] -> w291
                          frame False {
                          }
                          frame True {
                          }
                        }
                      }
                      frame True {
                        n112 = case shown="True" w296 {
                          tunnel: [Run_states."Set Frequency" ("Run states") Run_states."Set Device" ("Run states")] -> w295
                          frame False {
                          }
                          frame True {
                          }
                        }
                      }
                    }
                  }
                  frame True {
                    n113 = case shown="True" w301 {
                      tunnel: w300 -> [w303 w307]
                      tunnel: [w302 w306] -> w299
                      frame False {
                        n114 = case shown="False" w303 {
                          tunnel: [Run_states."Set Frequency" ("Run states") Run_states."Set Power" ("Run states")] -> w302
                          frame False {
                          }
                          frame True {
                          }
                        }
                      }
                      frame True {
                        n115 = case shown="True" w307 {
                          tunnel: [Run_states."Set Frequency" ("Run states") Run_states."Done" ("Run states")] -> w306
                          frame False {
                          }
                          frame True {
                          }
                        }
                      }
                    }
                  }
                }
              }
              frame "Device -> Frequency -> Power" {
                n116 = case shown="False" w313 {
                  tunnel: w312 -> [w316 w324]
                  tunnel: w311 -> [w315 w323]
                  tunnel: [w314 w322] -> w310
                  frame False {
                    n117 = case shown="True" w316 {
                      tunnel: w315 -> [_ w319]
                      tunnel: [Run_states."Set Power" ("Run states") w318] -> w314
                      frame False {
                      }
                      frame True {
                        n118 = case shown="False" w319 {
                          tunnel: [Run_states."Set Frequency" ("Run states") Run_states."Set Device" ("Run states")] -> w318
                          frame False {
                          }
                          frame True {
                          }
                        }
                      }
                    }
                  }
                  frame True {
                    n119 = case shown="False" w324 {
                      tunnel: w323 -> [w326 _]
                      tunnel: [w325 Run_states."Set Power" ("Run states")] -> w322
                      frame True {
                        n120 = case shown="False" w326 {
                          tunnel: [Run_states."Set Frequency" ("Run states") Run_states."Done" ("Run states")] -> w325
                          frame False {
                          }
                          frame True {
                          }
                        }
                      }
                      frame False {
                      }
                    }
                  }
                }
              }
            }
            n121 = flat-sequence {
              tunnel: w273 -> [w333]
              tunnel: [w333] -> w272
              tunnel: ["Cancel Button"] -> w268
              tunnel: [w331] -> w242
              tunnel: [w330] -> w241
              frame #0 {
                n122 = while {
                  shift-right: [w334] -> w330
                  shift-left: _ -> [w335]
                  tunnel: [w336] -> w331
                  stop <- TRUE stop-if-true
                  n123 = Get Date/Time In Seconds() -> (seconds since 1Jan1904=w334:timestamp)
                  n124 = Subtract(x=w334, y=w335) -> (x-y=w336:dbl)
                }
              }
            }
            n125 = call "Write XML Handler.lvclass.vi"("XML Handler.lvclass"=w276, "Measurements in"=w222) -> ("Measurements out"=w274:refnum<class "Harmonics.lvclass">)  [unwired: 9 in]
            n126 = Multiply(x=w243, y=w242) -> (x*y=w240:dbl)
            n127 = Add(x=w241, y=w240) -> (x+y=→"Estimated finish time":timestamp)
            n128 = Select(t=Run_states."Done", s=w268, f=w267) -> (s? t:f=w265:T3)
          }
          frame "Done" {
            n129 = call "Read PathControl.lvclass.vi"("Measurements in"=w342) -> ("PathControl.lvclass"=w344:refnum<class "PathControl.lvclass">)  [unwired: 9 in, 1 out]
            n130 = call "Read Frequency.vi"("Harmonics in"=w342) -> ("Frequency"=w348:cluster{"List":dbl[], "Index":i32, "Last":bool})  [unwired: 9 in, 1 out]
            n131 = call "Read Signal Generator.lvclass.vi"("Harmonics in"=w342) -> ("Signal Generator.lvclass"=w355:refnum<class "Signal Generator.lvclass">, "Harmonics out"=w364:refnum<class "Harmonics.lvclass">)  [unwired: 9 in]
            n132 = call "Read Power.vi"("Harmonics in"=w342) -> ("Power"=w352:cluster{"List":dbl[], "Index":i32, "Last":bool})  [unwired: 9 in, 1 out]
            n133 = Unbundle By Name(w348) -> ("List"=w347:dbl[], "Index"=w346:i32)
            n134 = Unbundle By Name(w352) -> ("List"=w339:dbl[])
            n135 = Decrement(x=w346) -> (x-1=w345:i32)
            n136 = Index Array(array=w347, index=w345) -> (element=w343:dbl)
            n137 = Array Max & Min(array=w339) -> (min value=w338:dbl)  [unwired: 3 out]
            n138 = call "Get Path Loss.vi"("Path"=Paths."SigGen 1 -> DUT", "Frequency [Hz]"=w343, "PathControl in"=w344) -> ("Insertion Loss (dB)"=w341:dbl)  [unwired: 5 in, 3 out]
            n139 = Subtract(x=w338, y=w341) -> (x-y=w340:dbl)
            n140 = call-dynamic "Configure Output Power.vi"("Output Power [dBm]"=w340, "Signal Generator in"=w355) -> ("error out"=w353:errorcluster, "Signal Generator out"=w354:refnum<class "Signal Generator.lvclass">)  [unwired: 8 in]
            n141 = call "Read Spectrum Analyzer.lvclass.vi"("Harmonics in"=w364) -> ("Spectrum Analyzer.lvclass"=w361:refnum<class "Spectrum Analyzer.lvclass">)  [unwired: 9 in, 1 out]
            n142 = call-dynamic "Enable Output.vi"("error in (no error)"=w353, "Output Enable (F)"=FALSE, "Signal Generator in"=w354) -> ("error out"=w362:errorcluster, "Signal Generator out"=w363:refnum<class "Signal Generator.lvclass">)  [unwired: 7 in]
            n143 = call-dynamic "Close Instrument.vi"("error in (no error)"=w362, "Instrument in"=w363) -> ("error out"=w358:errorcluster)  [unwired: 8 in, 1 out]
            n144 = call "Read Power Meter.lvclass.vi"("Harmonics in"=w342) -> ("Power Meter classes"=w351:refnum<class "Power Meter.lvclass">[])  [unwired: 9 in, 1 out]
            n145 = call-dynamic "Close Instrument.vi"("Instrument in"=w361) -> ("error out"=w359:errorcluster)  [unwired: 9 in, 1 out]
            n146 = for {
              tunnel: w351 -> [w374] mode=indexing
              tunnel: [w373] -> w356 mode=indexing
              n147 = call-dynamic "Close Instrument.vi"("Instrument in"=w374) -> ("error out"=w373:errorcluster)  [unwired: 9 in, 1 out]
            }
            n148 = Merge Errors(w360, w359, w358, w356) -> (w357:errorcluster)
          }
        }
      }
      frame Error {
      }
    }
  }
  "error out" <- w12
  "Harmonics out" <- w13
  "Canceled" <- w8
  "Parameters" <- w7
